vi "Format Error for Display.vi"(8 "error in (no error)":errorcluster, 11 "Error from Listbox":string) -> (0 "error out":errorcluster, 3 "Error formatted":string)   [LabVIEW 2026, in "TALOS.lvlib" / "Common GUI v3.lvlib" / "Common GUI v3.lvclass"]
uses:
  Common GUI v3.lvclass
  <vilib>/Utility/error.llb/Trim Whitespace (string).vi
  <vilib>/Utility/error.llb/Trim Whitespace One-Sided.vi
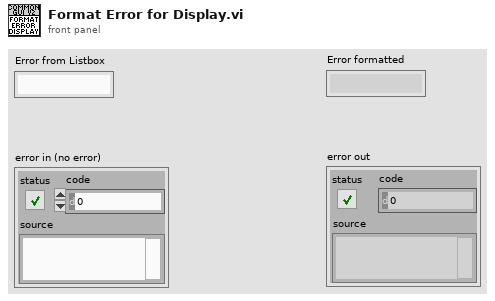
[diagram p1: front panel]
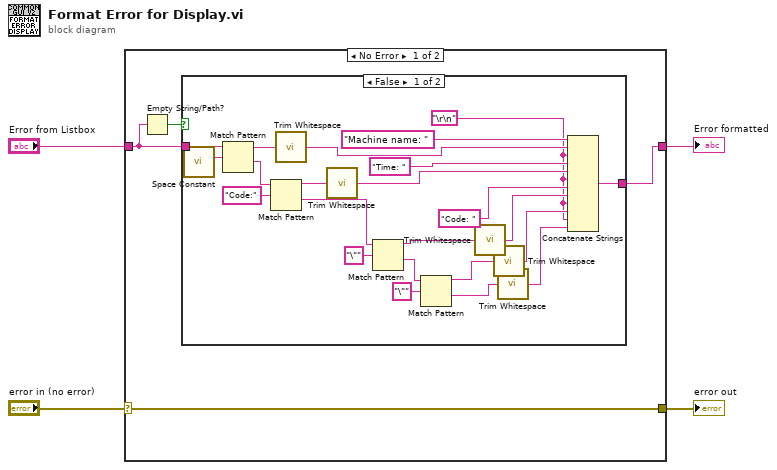
[diagram p0: block diagram]
diagram:
  n1 = case shown="No Error" "error in (no error)" {
    selector: "error in (no error)" -> [w7 w34]
    tunnel: "Error from Listbox" -> [w6 w33]
    tunnel: [w7 w34] -> w2
    tunnel: [w8 w33] -> w1
    frame No Error {
      n2 = Empty String/Path?(string/path=w6) -> (empty?=w5:bool)
      n3 = case shown="False" w5 {
        tunnel: [w14 w32] -> w8
        tunnel: w6 -> [w13 w32]
        frame False {
          w10 = "\r\n"
          n4 = call <vilib>:"Space Constant.vi"() -> ("String"=w31:string)
          n5 = Match Pattern(string=w13, regular expression=w31) -> (before substring=w29:string, after substring=w28:string)  [unwired: 1 in, 2 out]
          n6 = Match Pattern(string=w28, regular expression="Code:") -> (before substring=w12:string, after substring=w9:string)  [unwired: 1 in, 2 out]
          n7 = call-poly <vilib>:"Trim Whitespace.vi"("string"=w29) -> ("trimmed string"=w25:string)  [unwired: 1 in]
          n8 = call-poly <vilib>:"Trim Whitespace.vi"("string"=w12) -> ("trimmed string"=w11:string)  [unwired: 1 in]
          n9 = Match Pattern(string=w9, regular expression="\"") -> (before substring=w22:string, after substring=w19:string)  [unwired: 1 in, 2 out]
          n10 = Match Pattern(string=w19, regular expression="\"") -> (before substring=w18:string, after substring=w16:string)  [unwired: 1 in, 2 out]
          n11 = call-poly <vilib>:"Trim Whitespace.vi"("string"=w22) -> ("trimmed string"=w21:string)  [unwired: 1 in]
          n12 = call-poly <vilib>:"Trim Whitespace.vi"("string"=w18) -> ("trimmed string"=w17:string)  [unwired: 1 in]
          n13 = call-poly <vilib>:"Trim Whitespace.vi"("string"=w16) -> ("trimmed string"=w15:string)  [unwired: 1 in]
          n14 = Concatenate Strings("Machine name: " ("string"), w25, w10, "Time: " ("string"), w11, w10, "Code: " ("regular expression"), w21, w10, w17, w10, w15) -> (w14:string)
        }
        frame True {
        }
      }
    }
    frame Error {
    }
  }
  "Error formatted" <- w1
  "error out" <- w2
